vi "Manual Turret.vi"(10 "Enum":enum16{"Nothing", "Left", "Right"}(ring)) -> ()   [LabVIEW 2019]
uses:
  <vilib>/Rock Robotics/WPI/ThirdParty/Phoenix-LabVIEW/Motor Controller/Controls/CTRE_Phoenix_MotorControl_ControlMode.ctl
  max2020/RoboRIO/Refnums.vi
  <vilib>/Rock Robotics/WPI/ThirdParty/Phoenix-LabVIEW/Motor Controller/Get/CTRE_Phoenix_MotorController_GetQuadratureData.vi
  max2020/RoboRIO/Global Data.vi
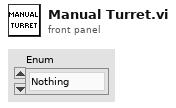
[diagram p1: front panel]
types:
  T1 = typedef "CTRE_Phoenix_MotorControl_ControlMode.ctl" = u16
  T2 = typedef "WPI_RobotDriveDevRef.ctl" = cluster{"DevStatus":errorcluster, "Motors[]":T3[], "Square Inputs":bool, "Max Output":dbl}
  T3 = typedef "WPI_MotorControlDeviceRef.ctl" = cluster{"DeviceStatus":errorcluster, "Type":T4, "PWM":cluster{"PWM Channel":T5, "DeadBand":T6}, "CAN":cluster{"Device Number":u8, "SetOutput VI Ref":variant, "GetOutput VI Ref":variant, "Enable VI Ref":variant, "Disable VI Ref":variant, "Data":variant}, "Invert":bool, "DIO PWM":cluster{"PWM \"Enable\" Channel":T5, "DIOChannel":T7, "PWM Rate":dbl}}
  T4 = typedef "WPI_MotorControlType.ctl" = enum16{"PWM", "CAN", "DIO PWM"}
  T5 = typedef "FPGA_DIOPWMChannel.ctl" = enum8{"PWM 0", "PWM 1", "PWM 2", "PWM 3", "PWM 4", "PWM 5", "PWM 6", "PWM 7", "PWM 8", "PWM 9", "PWM MXP 0", "PWM MXP 1", "PWM MXP 2", "PWM MXP 3", "PWM MXP 4", "PWM MXP 5", "PWM MXP 6", "PWM MXP 7", "PWM MXP 8", "PWM MXP 9", "Invalid"}
  T6 = typedef "WPI_PWMDeadband.ctl" = cluster{"Name":string, "maxPositivePwm":i32, "minPositivePwm":i32, "centerPwm":i32, "maxNegativePwm":i32, "minNegativePwm":i32, "angularRange":u16}
  T7 = typedef "FPGA_DIOChannel.ctl" = enum8{"DIO 0", "DIO 1", "DIO 2", "DIO 3", "DIO 4", "DIO 5", "DIO 6", "DIO 7", "DIO 8", "DIO 9", "DIO MXP 0", "DIO MXP 1", "DIO MXP 2", "DIO MXP 3", "DIO MXP 4", "DIO MXP 5", "DIO MXP 6", "DIO MXP 7", "DIO MXP 8", "DIO MXP 9", "DIO MXP 10", "DIO MXP 11", "DIO MXP 12", "DIO MXP 13", "DIO MXP 14", "DIO MXP 15", "SPI Port CS1", "SPI Port CS2", "SPI Port CS3", "SPI Port MISO", "SPI Port MOSI", "Invalid"}
  T8 = cluster{"ROBOT_DRIVE":T2, "RIGHT_DRIVE":T3, "LEFT_DRIVE":T3, "TURRET":T3, "SHOOTER_MASTER":T3, "HOPPER":T3, "INDEXER":T3, "INTAKE":T3, "CLIMBER_WINCH":T3, "CLIMBER_ARM":T3, "SHOOTER_ANGLE":T3, "SHOOTER_SLAVE":T3, "AGITATOR":T3, "AGITATOR OLD":T3}
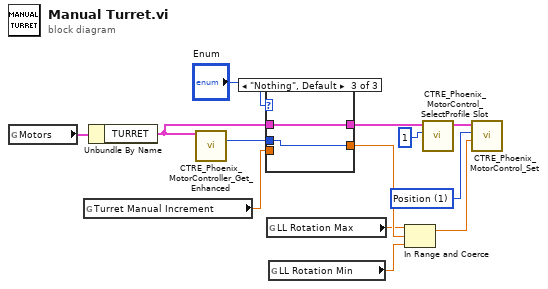
[diagram p0: block diagram]
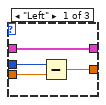
[diagram p2: hidden frame]
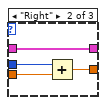
[diagram p3: hidden frame]
diagram:
  w10 = T1 1 items=["PercentOutput"=0, "Position"=1, "Velocity"=2, "Current"=3, "Follower"=5, "MotionProfile"=6, "MotionMagic"=7, "MotionProfileArc"=10, "Disabled"=15] ("Control Mode")
  n1 = global read "Refnums.vi" "Motors"() -> (w13:T8)
  n2 = global read "Global Data.vi" "Turret Manual Increment"() -> (w4:dbl)
  n3 = Unbundle By Name(w13) -> ("TURRET"=w12:T3)
  n4 = call-poly <vilib>:"CTRE_Phoenix_MotorController_Get_Enhanced.vi"("PhoenixMotorControlDevRef"=w12) -> ("Quadrature Position"=w11:i32)  [unwired: 11 in, 3 out]
  n5 = case shown="\"Nothing\", Default" "Enum" {
    tunnel: w12 -> [w14 w21 w23]
    tunnel: [w14 w21 w23] -> w9
    tunnel: w11 -> [w17 w19 w22]
    tunnel: [w15 w20 w22] -> w6
    tunnel: w4 -> [w16 w18 _]
    frame "Left" {
      n6 = Subtract(x=w17, y=w16) -> (x-y=w15:dbl)
    }
    frame "Right" {
      n7 = Add(x=w19, y=w18) -> (x+y=w20:dbl)
    }
    frame "Nothing", Default {
    }
  }
  n8 = global read "Global Data.vi" "LL Rotation Max"() -> (w2:dbl)
  n9 = global read "Global Data.vi" "LL Rotation Min"() -> (w1:dbl)
  n10 = In Range and Coerce(upper limit=w2, x=w6, lower limit=w1) -> (coerced(x)=w5:dbl)  [unwired: 1 out]
  n11 = call <vilib>:"CTRE_Phoenix_MotorControl_SelectProfile Slot.vi"("slotIdx"=1, "PhoenixMotorControlDevRef"=w9) -> ("PhoenixMotorControlDevRef"=w7:T3)  [unwired: 8 in, 1 out]
  n12 = call <vilib>:"CTRE_Phoenix_MotorControl_Set.vi"("Output"=w5, "Control Mode"=w10, "PhoenixMotorControlDevRef"=w7) -> ()  [unwired: 7 in, 2 out]
